vi "FVIR_LDO_LongCycleCheck.vi"(11 "Total Cycle Counter":u16) -> (3 "Short Cycle?":bool)   [LabVIEW 2020]
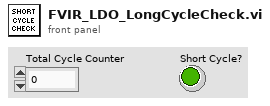
[diagram p1: front panel]
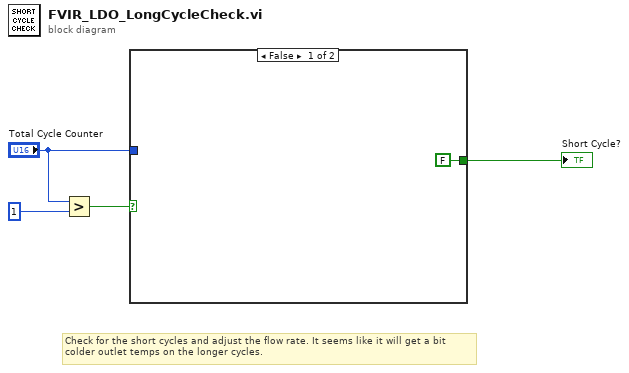
[diagram p0: block diagram]
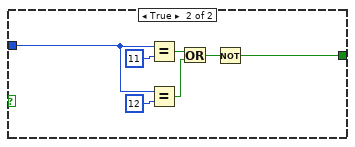
[diagram p2: hidden frame]
diagram:
  # "Check for the short cycles and adjust the flow rate. It seems like it will get a bit\ncolder outlet temps on the longer cycles."
  n1 = Greater?(x="Total Cycle Counter", y=u16 1) -> (0:w1:bool)
  n2 = case shown="False" w1 {
    tunnel: [FALSE w7] -> w4
    tunnel: "Total Cycle Counter" -> [_ w6]
    frame False {
    }
    frame True {
      n3 = Equal?(x=w6, y=u16 11) -> (x = y?=w11:bool)
      n4 = Equal?(x=w6, y=u16 12) -> (x = y?=w12:bool)
      n5 = Or(x=w11, y=w12) -> (x .or. y?=w8:bool)
      n6 = Not(x=w8) -> (.not. x?=w7:bool)
    }
  }
  "Short Cycle?" <- w4
